vi "Get 1 Pin Information.vi"(8 "error in":errorcluster, 10 "pin or relay name":string, 11 "session reservation in":refnum<class "Session Reservation.lvclass">) -> (0 "error out":errorcluster, 1 "pin instrument":refnum<class>, 2 "channel_mappings":T1, 3 "session reservation our":refnum<class "Session Reservation.lvclass">)   [LabVIEW 2021, in "Get Pin Information.lvlib"]
uses:
  Get Pin Information.lvlib
  <vilib>/Plug-In SDKs/Clients/Session Management V1/Session Reservation/Session Reservation.lvclass
  <vilib>/gRPC/Generated APIs/ni/measurementlink/sessionmanagement/v1/RPC Messages/ni_measurementlink_sessionmanagement_v1_ChannelMapping.ctl
  <vilib>/Plug-In SDKs/Clients/Session Management V1/Session Reservation/Session Reservation.lvclass/Session Reservation.ctl
  <vilib>/Plug-In SDKs/Clients/Session Management V1/Session Reservation/Get Session Info - 1Sess .vi
  <vilib>/Plug-In SDKs/Clients/Session Management V1/Session Reservation/Get Session Info - NSess .vi
  <vilib>/Plug-In SDKs/Clients/Session Management V1/Session Reservation/Merge Invalid DVR Error.vi
  <vilib>/Plug-In SDKs/Clients/Session Management V1/Session Reservation/Is DVR Valid.vi
  <vilib>/Plug-In SDKs/Measurements/Helpers/Error Strings Global Internal.vi
  <vilib>/Utility/error.llb/Error Cluster From Error Code.vi
  <vilib>/gRPC/Generated APIs/ni/measurementlink/sessionmanagement/v1/ni.measurementlink.sessionmanagement.v1.api.lvlib
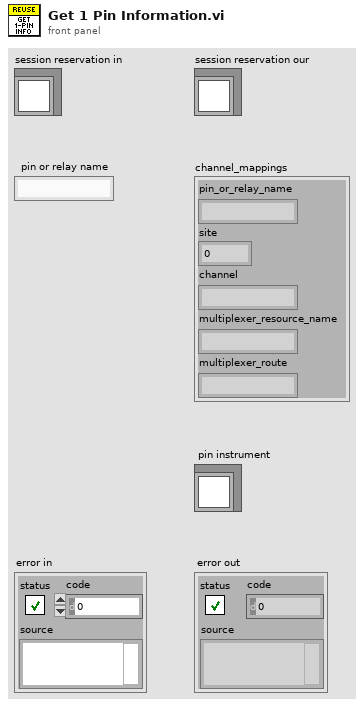
[diagram p1: front panel]
types:
  T1 = typedef "ni.measurementlink.sessionmanagement.v1.api.lvlib/ni_measurementlink_sessionmanagement_v1_ChannelMapping.ctl" = cluster{"pin_or_relay_name":string, "site":i32, "channel":string, "multiplexer_resource_name":string, "multiplexer_route":string}
  T2 = typedef "ni.measurementlink.sessionmanagement.v1.api.lvlib/ni_measurementlink_sessionmanagement_v1_SessionInformation.ctl" = cluster{"session":T3, "resource_name":string, "channel_list":string, "instrument_type_id":string, "session_exists":bool, "channel_mappings":T1[]}
  T3 = typedef "ni.measurementlink.sessionmanagement.v1.api.lvlib/nidevice_grpc_Session.ctl" = cluster{"name":string}
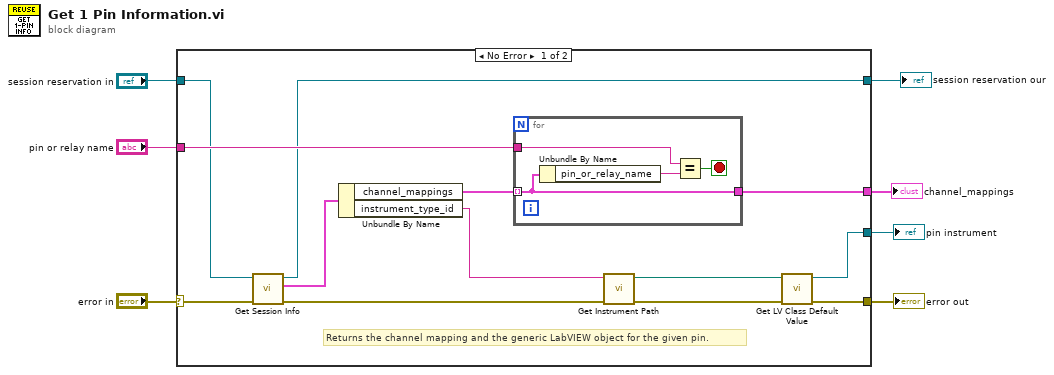
[diagram p0: block diagram]
diagram:
  n1 = case shown="No Error" "error in" {
    selector: "error in" -> [w17 w26]
    tunnel: "pin or relay name" -> [w18 _]
    tunnel: [w16 w26] -> w5
    tunnel: [w15 _] -> w4
    tunnel: [w10 w25] -> w3
    tunnel: "session reservation in" -> [w9 w25]
    tunnel: [w8 _] -> w1
    frame No Error {
      # "Returns the channel mapping and the generic LabVIEW object for the given pin."
      n2 = call-poly <vilib>:"Get Session Info.vi"("error in"=w17, "session reservation in"=w9) -> ("error out"=w12:errorcluster, "session info"=w20:T2, "session reservation out"=w10:refnum<class "Session Reservation.lvclass">)  [unwired: 7 in]
      n3 = Unbundle By Name(w20) -> ("channel_mappings"=w19:T1[], "instrument_type_id"=w13:string)
      n4 = for {
        tunnel: w19 -> [w21] mode=indexing
        tunnel: w18 -> [w24]
        tunnel: [w21] -> w8
        stop <- w22 stop-if-true
        n5 = Unbundle By Name(w21) -> ("pin_or_relay_name"=w23:string)
        n6 = Equal?(x=w24, y=w23) -> (x = y?=w22:bool)
      }
      n7 = call "Get Instrument Path.vi"("error in"=w12, "instrument_type_id"=w13) -> ("error out"=w11:errorcluster, "Instrument Path"=w14:path)  [unwired: 8 in]
      n8 = call <vilib>:"Get LV Class Default Value.vi"("error in (no error)"=w11, "class path"=w14) -> ("error out"=w16:errorcluster, "object"=w15:refnum<class>)  [unwired: 8 in]
    }
    frame Error {
    }
  }
  "error out" <- w5
  "pin instrument" <- w4
  "session reservation our" <- w3
  "channel_mappings" <- w1
